vi "CtrlCmdCreator.vi"(1 "dt":string, 2 "acid":string, 3 "rq":dbl, 4 "cmd":string) -> (0 "JSON字符串":string)   [LabVIEW 2016]
panel:
  # "command，命令类型"
  # "接收命令的CtrlAccsory的ID"
  # "实际传输的数据"
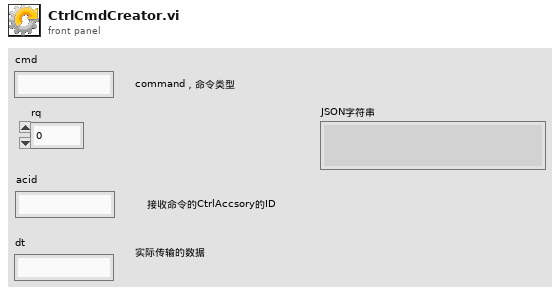
[diagram p1: front panel]
types:
  T1 = cluster{"cmd":string, "acid":string, "rq":dbl, "dt":string}
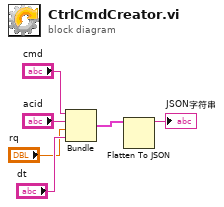
[diagram p0: block diagram]
diagram:
  n1 = Bundle("cmd"="cmd", "acid"="acid", "rq"="rq", "dt"="dt") -> (w3:T1)  [unwired: 1 in]
  n2 = Flatten To JSON(anything=w3) -> (JSON string=→"JSON字符串":string)  [unwired: 2 in, 1 out]
